vi "Lockin.listDependencies.vi"(8 "error in (no error)":errorcluster, 11 "Instrument.Lockin in":refnum<class "Instrument.Lockin.lvclass">) -> (0 "error out":errorcluster, 2 "Dependencies":T1, 3 "Instrument.Lockin out":refnum<class "Instrument.Lockin.lvclass">)   [LabVIEW 2019, in "Instrument.Lockin.lvlib" / "Instrument.Lockin.lvclass"]
uses:
  Instrument.Lockin.lvclass
  C:/Program Files (x86)/National Instruments/LabVIEW 2019/vi.lib/JKI/JKI SMO/SMO/SMO.lvclass
  Typedefs/Lockin.Dependencies--Cluster.ctl
  Instrument.DAQ/Instrument.DAQ.lvclass
  Instrument.Lockin.lvclass/Instrument.Lockin.ctl
  <vilib>/JKI/JKI SMO/SMO/SMO.lvclass
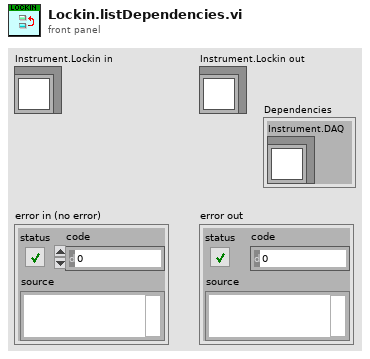
[diagram p1: front panel]
types:
  T1 = typedef "Instrument.Lockin.lvlib/Instrument.Lockin.lvclass/Lockin.Dependencies--Cluster.ctl" = cluster{"Instrument.DAQ":refnum<class "Instrument.DAQ.lvclass">}
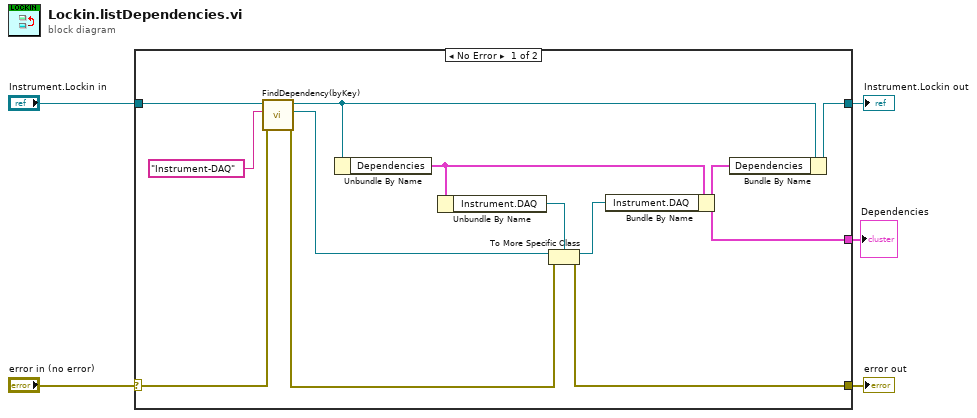
[diagram p0: block diagram]
diagram:
  n1 = case shown="No Error" "error in (no error)" {
    selector: "error in (no error)" -> [w14 w19]
    tunnel: [w15 w19] -> w5
    tunnel: [w13 w18] -> w3
    tunnel: "Instrument.Lockin in" -> [w11 w18]
    tunnel: [w6 _] -> w1
    frame No Error {
      n2 = call <vilib>:"FindDependency(byKey).vi"("error in (no error)"=w14, "Key"="Instrument-DAQ", "SMO in"=w11) -> ("error out"=w16:errorcluster, "Dependency"=w10:refnum<class "SMO.lvclass">, "SMO dup"=w12:refnum<class "Instrument.Lockin.lvclass">)  [unwired: 5 in, 1 out]
      n3 = Unbundle By Name(w12) -> ("Dependencies"=w8:T1)
      n4 = Unbundle By Name(w8) -> ("Instrument.DAQ"=w7:refnum<class "Instrument.DAQ.lvclass">)
      n5 = To More Specific Class(target class=w7, reference=w10, error in=w16) -> (specific class reference=w17:refnum<class "Instrument.DAQ.lvclass">, error out=w15:errorcluster)
      n6 = Bundle By Name(cluster=w8, "Instrument.DAQ"=w17) -> (w6:T1)
      n7 = Bundle By Name(cluster=w12, "Dependencies"=w6) -> (w13:refnum<class "Instrument.Lockin.lvclass">)
    }
    frame Error {
    }
  }
  "error out" <- w5
  "Instrument.Lockin out" <- w3
  "Dependencies" <- w1
